vi "Balance Inquiry.vi"(8 "error in (no error)":errorcluster, 11 "Module Data":T1) -> (0 "error out":errorcluster, 3 "Balance":string)   [LabVIEW 2016]
doc: "Determines balance as per account number provided."
uses:
  Controls/UI Controls.ctl
  Controls/ATM Messages.ctl
  Controls/Module Data.ctl
  Controls/User Input Data.ctl
  Controls/Transaction Status.ctl
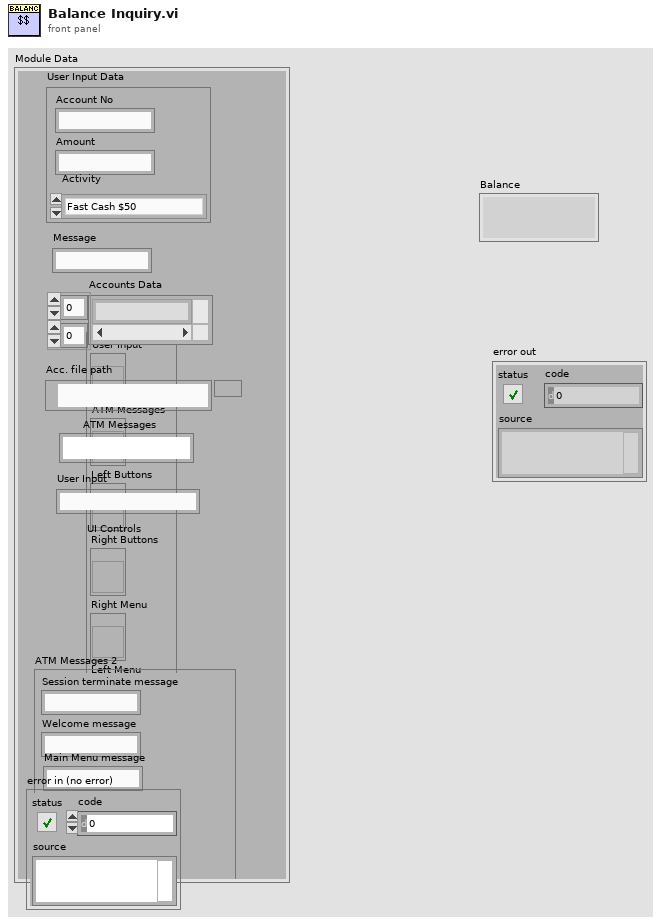
[diagram p1: front panel]
types:
  T1 = typedef "Module Data.ctl" = cluster{"UI Controls":T2, "ATM Messages 2":T3, "User Input":string, "ATM Messages":string, "Acc. file path":path, "Accounts Data":string[][], "User Input Data":T4, "Message":string}
  T2 = typedef "UI Controls.ctl" = cluster{"ATM Messages":refnum<vi>, "User Input":refnum<vi>, "Right Buttons":refnum<vi>, "Right Menu":refnum<vi>, "Left Buttons":refnum<vi>, "Left Menu":refnum<vi>, "Card Simulator":refnum<vi>, "Enter":refnum<vi>}
  T3 = typedef "ATM Messages.ctl" = cluster{"Session terminate message":string, "Welcome message":string, "Deposit Message":string, "Deposit Complete Message":string, "Withdrawal Message":string, "Withdrawal Complete Message":string, "Balance Inquiry Message":string, "Account verification failed message":string, "Withdrawal failed message":string, "Card Inserted":string, "Main Menu message":string}
  T4 = typedef "User Input Data.ctl" = cluster{"Account No":string, "Amount":string, "Activity":T5}
  T5 = typedef "Transaction Status.ctl" = enum16{"Fast Cash $50", "Withdrawal?", "Deposit?", "Account Number?"}
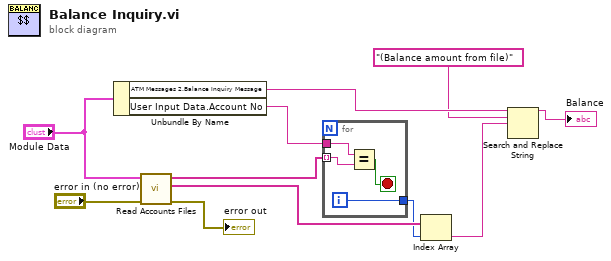
[diagram p0: block diagram]
diagram:
  n1 = Unbundle By Name("Module Data") -> ("ATM Messages 2.Balance Inquiry Message"=w4:string, "User Input Data.Account No"=w10:string)
  n2 = call "Read Accounts Files.vi"("error in (no error)"="error in (no error)", "Module Data"="Module Data") -> ("error out"=→"error out":errorcluster, "Balances Column"=w9:string[], "Acc Numbers Column"=w7:string[])  [unwired: 6 in, 1 out]
  n3 = for {
    tunnel: w10 -> [w13]
    tunnel: w7 -> [w14] mode=indexing
    tunnel: [w12] -> w8
    i -> [w12]
    stop <- w15 stop-if-true
    n4 = Equal?(x=w13, y=w14) -> (x = y?=w15:bool)
  }
  n5 = Index Array(array=w9, index=w8) -> (element=w2:string)
  n6 = Search and Replace String(input string=w4, search string="(Balance amount from file)" ("replace string (\"\")"), replace string=w2) -> (result string=→"Balance":string)  [unwired: 5 in, 3 out]
